vi "QPSK.vi"() -> ()   [LabVIEW 2019]
uses:
  <vilib>/measure/madcrms.llb/Basic Averaged DC-RMS for N Chan.vi
  <vilib>/Analysis/NI_AALBase.lvlib
  <vilib>/measure/NI_MAPro.lvlib
panel:
  out "output graph":dbl[](graph)
  out "input graph":dbl[](graph)
  out "input bits":dbl[](array[numeric])
  out "output bits":dbl[](array[numeric])
  out "Constellation Graph(Reciever)":cluster{"Y":dbl[], "Y":dbl[]}[](graph)
  out "odd de part":dynamicdata(graph)
  out "even de part":dynamicdata(graph)
  in  "standard deviation":dbl=1.0000000000000002 format="%0.2f"
  out "odd part":dynamicdata(graph)
  out "even part":dynamicdata(graph)
  out "Transmitting wave":dynamicdata(graph)
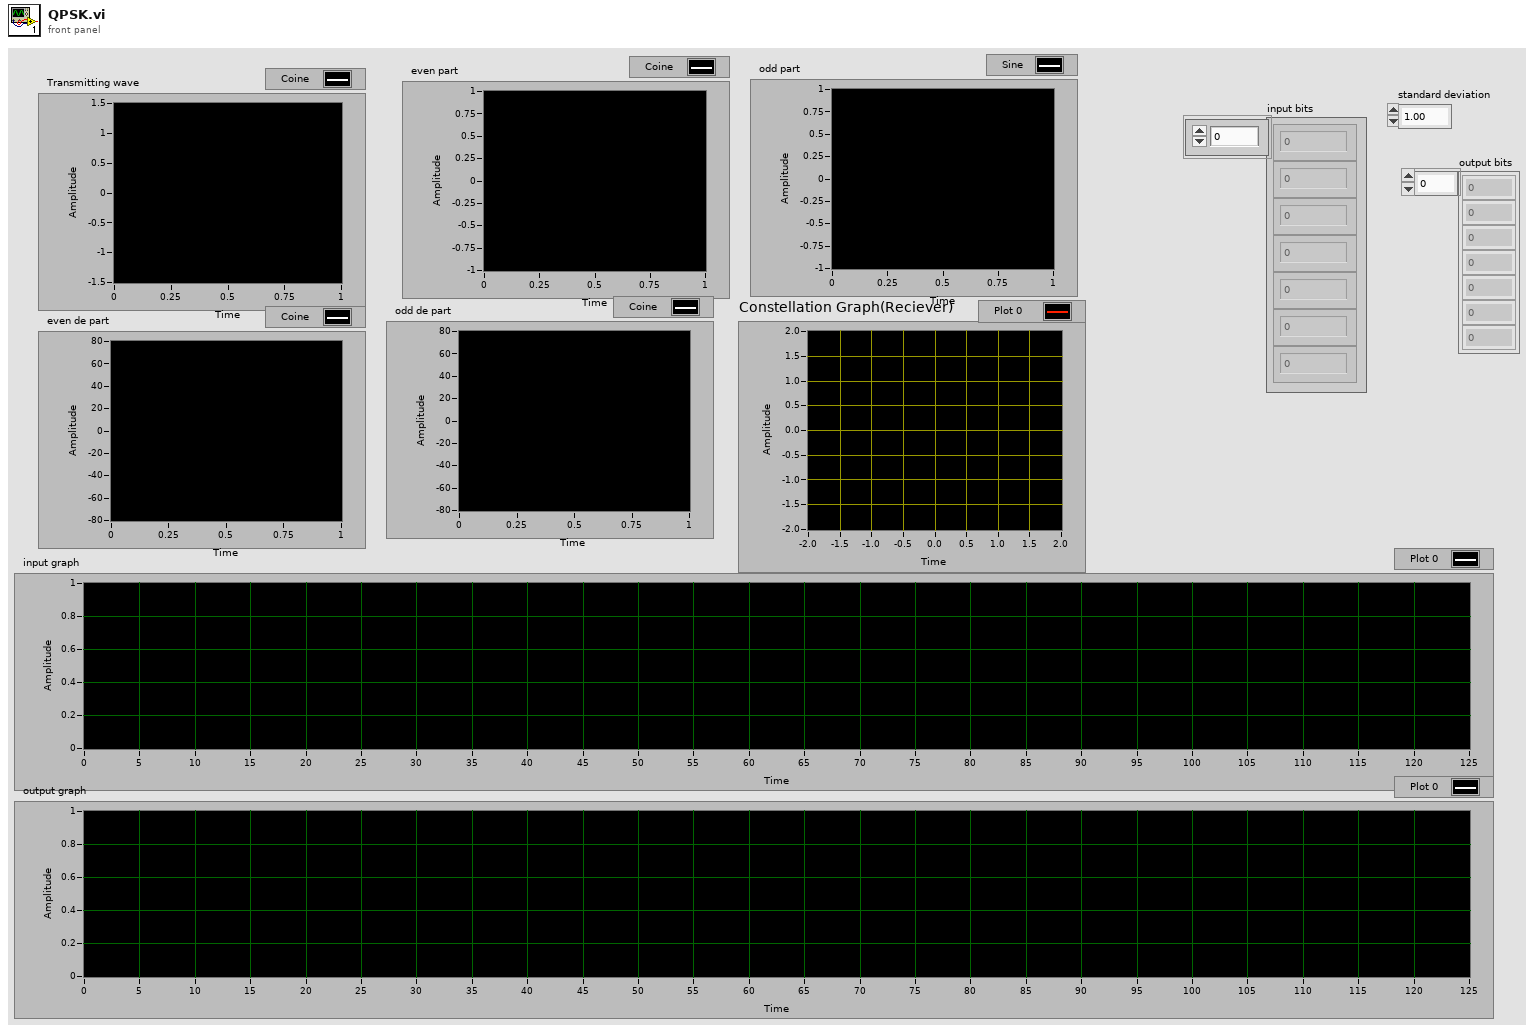
[diagram p1: front panel]
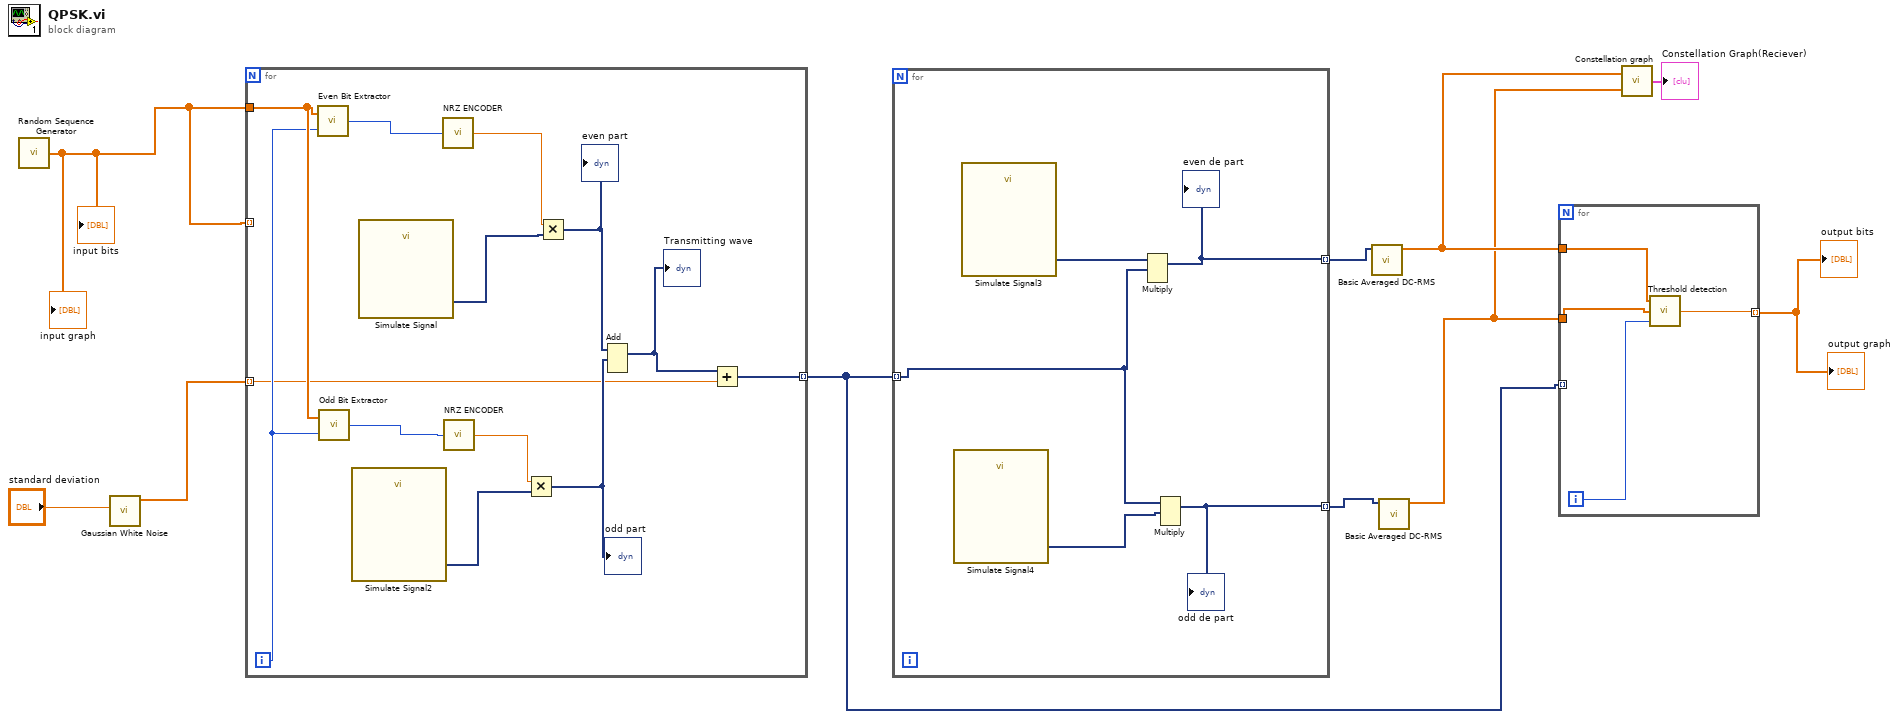
[diagram p0: block diagram]
diagram:
  n1 = call "Random Sequence Generator.vi"() -> ("Array"=w2:dbl[])
  "input bits" <- w2
  "input graph" <- w2
  n2 = call <vilib>:"Gaussian White Noise.vi"("standard deviation"="standard deviation") -> ("Gaussian noise pattern"=w9:dbl[])  [unwired: 9 in, 1 out]
  n3 = for {
    tunnel: w2 -> [w23]
    tunnel: w9 -> [w13] mode=indexing
    tunnel: [w12] -> w3 mode=indexing
    tunnel: w2 -> [_] mode=indexing
    i -> [w22]
    n4 = call "Even Bit Extractor.vi"("Loop Index"=w22, "Input PN Sequence"=w23) -> ("Even Bits"=w21:i8)
    n5 = call "Odd Bit Extractor.vi"("Loop Index"=w22, "Input PN Sequence"=w23) -> ("Odd Bits"=w20:i8)
    n6 = call "Simulate Signal2"() -> ("Sine"=w16:dynamicdata)  [unwired: 14 in, 1 out]
    n7 = call "Simulate Signal"() -> ("Coine"=w18:dynamicdata)  [unwired: 14 in, 1 out]
    n8 = call "NRZ ENCODER.vi"("Input Bit"=w21) -> ("NRZ Output"=w19:dbl)
    n9 = call "NRZ ENCODER.vi"("Input Bit"=w20) -> ("NRZ Output"=w17:dbl)
    n10 = Multiply(x=w17, y=w16) -> (x*y=w14:dynamicdata)
    "odd part" <- w14
    n11 = Multiply(x=w19, y=w18) -> (x*y=w15:dynamicdata)
    "even part" <- w15
    n12 = Add(1:w14, 2:w15) -> (0:w11:dynamicdata)  [unwired: 1 in, 1 out]
    "Transmitting wave" <- w11
    n13 = Add(x=w11, y=w13) -> (x+y=w12:dynamicdata)
  }
  n14 = for {
    tunnel: w3 -> [w25] mode=indexing
    tunnel: [w28] -> w8 mode=indexing
    tunnel: [w27] -> w7 mode=indexing
    n15 = call "Simulate Signal4"() -> ("Sine"=w24:dynamicdata)  [unwired: 14 in, 1 out]
    n16 = call "Simulate Signal3"() -> ("Coine"=w26:dynamicdata)  [unwired: 14 in, 1 out]
    n17 = Multiply(1:w25, 2:w26) -> (0:w28:dynamicdata)  [unwired: 1 in, 1 out]
    "even de part" <- w28
    n18 = Multiply(1:w24, 2:w25) -> (0:w27:dynamicdata)  [unwired: 1 in, 1 out]
    "odd de part" <- w27
  }
  n19 = call-poly <vilib>:"Basic Averaged DC-RMS.vi"("signals in"=w8) -> ("DC values"=w6:dbl[])  [unwired: 7 in, 3 out]
  n20 = call-poly <vilib>:"Basic Averaged DC-RMS.vi"("signals in"=w7) -> ("DC values"=w5:dbl[])  [unwired: 7 in, 3 out]
  n21 = for {
    tunnel: w6 -> [w32]
    tunnel: w5 -> [w31]
    tunnel: [w29] -> w1 mode=indexing
    tunnel: w3 -> [_] mode=indexing
    i -> [w30]
    n22 = call "Threshold detection.vi"("index"=w30, "f"=w31, "t"=w32) -> ("Output"=w29:dbl)
  }
  "output bits" <- w1
  "output graph" <- w1
  n23 = call "Constellation graph.vi"("Odd Bits"=w5, "Even Bits"=w6) -> ("Constellation Graph(Reciever)"=→"Constellation Graph(Reciever)":cluster{"Y":dbl[], "Y":dbl[]}[])
